vi "1D Indicator.vi"(10 "Color":u32(colorbox)=6618880, 11 "Numeric Value":u8) -> (3 "Raw Data":u8[](array[numeric]))   [LabVIEW 2019, in "LED Matrix Host.lvlib"]
uses:
  LED Matrix Host.lvlib
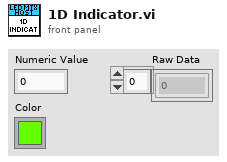
[diagram p1: front panel]
types:
  T1 = typedef "LED Matrix Host.lvlib/Frame.ctl" = cluster{"Matrix":u32[][]}
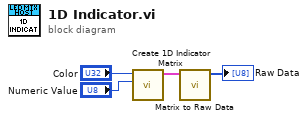
[diagram p0: block diagram]
diagram:
  n1 = call "Create 1D Indicator Matrix.vi"("Numeric Value"="Numeric Value", "Color"="Color") -> ("Matrix"=w1:T1)  [unwired: 9 in]
  n2 = call "Matrix to Raw Data.vi"("Matrix"=w1) -> ("Raw Data"=→"Raw Data":u8[])  [unwired: 10 in]
